vi "Configure Date And Time.vi"(0 "VISA resource name":refnum<visa-resource-name>, 1 "Display Clock (T: Enable)":bool=TRUE, 5 "Year (2005)":i32=2005, 7 "Month (1)":i32=1, 9 "Day  (1)":i32=1, 11 "error in (no error)":errorcluster, 12 "Hour  (0)":i32, 13 "Minute (0)":i32, 14 "Second (0)":i32) -> (4 "VISA resource name out":refnum<visa-resource-name>, 15 "error out":errorcluster)   [LabVIEW 2018, in "Agilent ENA Series.lvlib"]
doc: "Configures date and time settings."
uses:
  Agilent ENA Series.lvlib
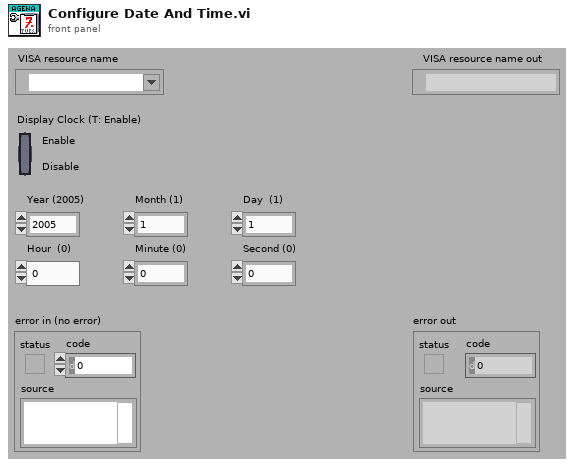
[diagram p1: front panel]
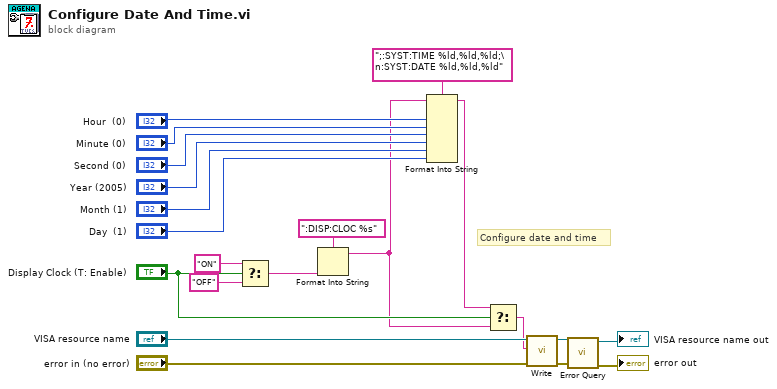
[diagram p0: block diagram]
diagram:
  # "Configure date and time"
  n1 = Select(t="ON", s="Display Clock (T: Enable)", f="OFF") -> (s? t:f=w16:string)
  n2 = Format Into String(format string=":DISP:CLOC %s", w16) -> (resulting string=w7:string)  [unwired: 2 in, 1 out]
  n3 = Format Into String(format string=";:SYST:TIME %ld,%ld,%ld;\n:SYST:DATE %ld,%ld,%ld", initial string=w7, "Hour  (0)", "Minute (0)", "Second (0)", "Year (2005)", "Month (1)", "Day  (1)") -> (resulting string=w6:string)  [unwired: 1 in, 1 out]
  n4 = Select(t=w6, s="Display Clock (T: Enable)", f=w7) -> (s? t:f=w5:string)
  n5 = call "Write.vi"("error in (no error)"="error in (no error)", "String ()"=w5, "VISA resource name"="VISA resource name") -> ("error out"=w3:errorcluster, "VISA resource name out"=w4:refnum<visa-resource-name>)  [unwired: 6 in, 1 out]
  n6 = call "Error Query.vi"("error in (no error)"=w3, "VISA resource name"=w4) -> ("error out"=→"error out":errorcluster, "VISA resource name out"=→"VISA resource name out":refnum<visa-resource-name>)  [unwired: 6 in, 2 out]
